vi "write_DACs.vi"(11 "DAC values in":T1 {"bit index" min=-1 max=17 step=1; "channel index" max=7 step=1; "offset" max=4095; "DAC voltage"."ch1" max=4095 step=1; "DAC voltage"."ch0" max=4095 step=1}) -> (3 "DAQ values out":T1 {"bit index" min=-1 max=17 step=1; "channel index" max=7 step=1; "offset" max=4095; "DAC voltage"."ch1" max=4095 step=1; "DAC voltage"."ch0" max=4095 step=1})   [LabVIEW 2011]
uses:
  typedefs/DAC_values_cluster.ctl
  typedefs/DAC_voltage_cluster.ctl
  <vilib>/rvi/eio/common/nirviEmuTemplateMethod_errors.vi
  <vilib>/eio/EIONode/EIONode.xnode
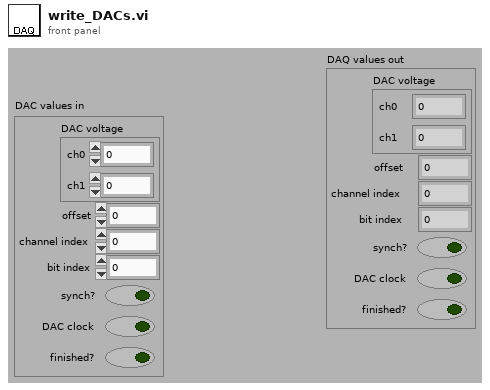
[diagram p1: front panel]
types:
  T1 = typedef "DAC_values_cluster.ctl" = cluster{"DAC voltage":T2, "offset":u16, "channel index":u16, "bit index":i32, "synch?":bool, "DAC clock":bool, "finished?":bool}
  T2 = typedef "DAC_voltage_cluster.ctl" = cluster{"ch0":u16, "ch1":u16}
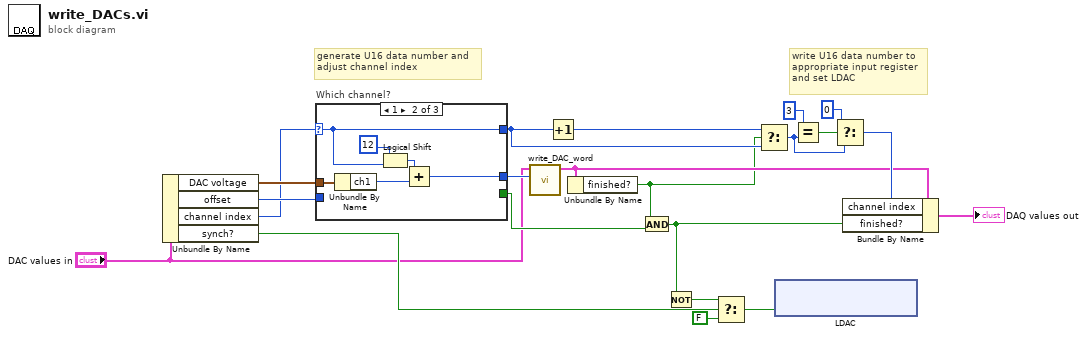
[diagram p0: block diagram]
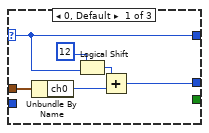
[diagram p2: hidden frame]
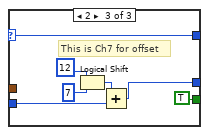
[diagram p3: hidden frame]
diagram:
  # "write U16 data number to\nappropriate input register\nand set LDAC"
  # "generate U16 data number and\nadjust channel index"
  n1 = Unbundle By Name("DAC values in") -> ("DAC voltage"=w10:T2, "offset"=w9:u16, "channel index"=w1:u16, "synch?"=w8:bool)
  n2 = case "Which channel?" shown="1" w1 {
    selector: w1 -> [w22 w28 w34]
    tunnel: w10 -> [w24 w33 _]
    tunnel: w9 -> [_ _ w38]
    tunnel: [w23 w29 w36] -> w21
    tunnel: [_ _ TRUE] -> w18
    tunnel: [w22 w28 w34] -> w16
    frame 0, Default {
      n3 = Unbundle By Name(w24) -> ("ch0"=w27:u16)
      n4 = Logical Shift(y=u16 12, x=w22) -> (x << y=w25:u16)
      n5 = Add(x=w25, y=w27) -> (x+y=w23:u16)
    }
    frame 1 {
      n6 = Unbundle By Name(w33) -> ("ch1"=w30:u16)
      n7 = Logical Shift(y=u16 12, x=w28) -> (x << y=w32:u16)
      n8 = Add(x=w32, y=w30) -> (x+y=w29:u16)
    }
    frame 2 {
      # "This is Ch7 for offset"
      n9 = Logical Shift(y=u16 12, x=u16 7) -> (x << y=w39:u16)
      n10 = Add(x=w39, y=w38) -> (x+y=w36:u16)
    }
  }
  n11 = call "write_DAC_word.vi"("U16 data number"=w21, "DAC values in"="DAC values in") -> ("DAC values out"=w3:T1)  [unwired: 9 in]
  n12 = Increment(x=w16) -> (x+1=w15:u16)
  n13 = Unbundle By Name(w3) -> ("finished?"=w2:bool)
  n14 = And(x=w2, y=w18) -> (x .and. y?=w7:bool)
  n15 = Not(x=w7) -> (.not. x?=w17:bool)
  n16 = Select(t=w17, s=w8, f=FALSE) -> (s? t:f=w19:bool)
  n17 = Select(t=w15, s=w2, f=w16) -> (s? t:f=w11:u16)
  n18 = xnode "LDAC"("Connector1/DIO32"=w19) -> ()  [unwired: 1 in, 1 out]
  n19 = Equal?(x=u16 3, y=w11) -> (x = y?=w13:bool)
  n20 = Select(t=u16 0, s=w13, f=w11) -> (s? t:f=w6:u16)
  n21 = Bundle By Name(cluster=w3, "channel index"=w6, "finished?"=w7) -> (→"DAQ values out":T1)
